vi "Query Channel Parameters.vi"(7 "Channel (1:Chan A)":i32(ring)=1 items=["Channel A"=1, "Channel B"=2, "Channel C"=3, "Channel D"=4, "Channel E"=5, "Channel F"=6, "Channel G"=7, "Channel H"=8], 8 "error in (no error)":errorcluster, 11 "VISA resource name":refnum<visa-resource-name>) -> (0 "error out":errorcluster, 2 "Chan Parameters":T1={"Channel"=1, "Chan State"=TRUE, "Chan Sync Source"=0, "Chan Gate Logic"=enum."Disabled", "Chan Mode"=enum."Normal", "Chan Wait #"=-1, "Chan Delay"=nan, "Chan Width"=nan, "Chan Burst #"=-1, "Chan DC On"=-1, "Chan DC Off"=-1, "Chan Polarity"=FALSE, "Chan MUX Value"=-1, "Chan Level Out"=enum."TTL", "Chan Lev Adjust"=0.0, "Chan Gate Mode"=enum."Disabled"} {"Chan Sync Source" items=["System (To)", "Channel A", "Channel B", "Channel C", "Channel D", "Channel E", "Channel F", "Channel G", "Channel H"]; "Chan Width" format="%.3p"; "Chan Delay" format="%.3p"; "Chan Lev Adjust" format="%.3p"; "Channel" items=["Channel A"=1, "Channel B"=2, "Channel C"=3, "Channel D"=4, "Channel E"=5, "Channel F"=6, "Channel G"=7, "Channel H"=8]}, 3 "VISA resource name out":refnum<visa-resource-name>)   [LabVIEW 2013]
doc: "This VI reads all channel parameters for the selected channel."
uses:
  Channel Parameters.ctl
  Berkeley Nucleonics 500 Series.lvlib
panel:
  # "Input"
  # "Normal\nSingle\nBurst"
  # "Burst"
  # "Duty Cycle"
  # "Output"
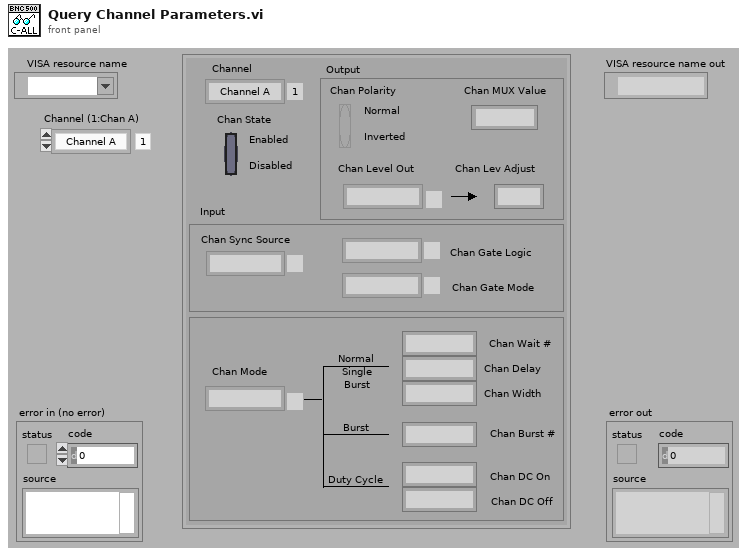
[diagram p1: front panel]
types:
  T1 = typedef "Channel Parameters.ctl" = cluster{"Channel":i32, "Chan State":bool, "Chan Sync Source":i32, "Chan Gate Logic":enum16{"Disabled", "Low", "High"}, "Chan Mode":enum16{"Normal", "Single", "Burst", "Duty Cycle"}, "Chan Wait #":i32, "Chan Delay":dbl, "Chan Width":dbl, "Chan Burst #":i32, "Chan DC On":i32, "Chan DC Off":i32, "Chan Polarity":bool, "Chan MUX Value":i32, "Chan Level Out":enum16{"TTL", "Adjustable", "35 Volt", "Optical"}, "Chan Lev Adjust":dbl, "Chan Gate Mode":enum16{"Disabled", "Pulse Inhibit", "Output Inhibit"}}
  T2 = cluster{"Gate Logic":enum16{"Disabled", "Low", "High"}, "Sync Source":i32, "Gate Mode":enum16{"Disabled", "Pulse Inhibit", "Output Inhibit"}}
  T3 = enum16{"Disabled", "Pulse Inhibit", "Output Inhibit"}
  T4 = cluster{"Mode":enum16{"Normal", "Single", "Burst", "Duty Cycle"}, "Burst #":i32, "DC Off":i32, "DC On":i32, "Delay":dbl, "Width":dbl, "Wait #":i32}
  T5 = enum16{"Normal", "Single", "Burst", "Duty Cycle"}
  T6 = cluster{"Polarity Out":bool, "Level Value":dbl, "Level Out":enum16{"TTL", "Adjustable", "35 Volt", "Optical"}, "MUX Value":i32}
  T7 = enum16{"TTL", "Adjustable", "35 Volt", "Optical"}
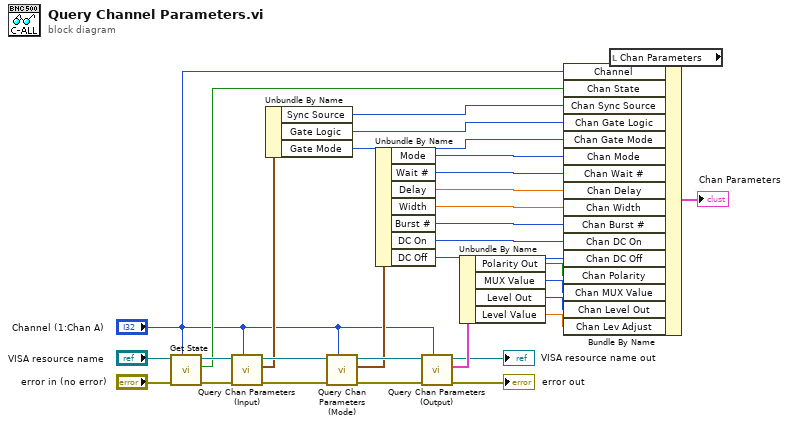
[diagram p0: block diagram]
diagram:
  n1 = call "Get State.vi"("Channel (1: Chan A)"="Channel (1:Chan A)", "error in (no error)"="error in (no error)", "VISA resource name"="VISA resource name") -> ("error out"=w26:errorcluster, "State"=w23:bool, "VISA resource name out"=w27:refnum<visa-resource-name>)  [unwired: 6 in]
  n2 = call "Query Chan Parameters (Input).vi"("Channel (1: Chan A)"="Channel (1:Chan A)", "error in (no error)"=w26, "VISA resource name"=w27) -> ("error out"=w30:errorcluster, "Input Parameters"=w22:T2, "VISA resource name out"=w31:refnum<visa-resource-name>)  [unwired: 6 in]
  n3 = Unbundle By Name(w22) -> ("Sync Source"=w21:i32, "Gate Logic"=w20:enum16{"Disabled", "Low", "High"}, "Gate Mode"=w2:T3)
  n4 = call "Query Chan Parameters (Mode).vi"("Channel (1: Chan A)"="Channel (1:Chan A)", "error in (no error)"=w30, "VISA resource name"=w31) -> ("error out"=w29:errorcluster, "Mode Parameters"=w19:T4, "VISA resource name out"=w28:refnum<visa-resource-name>)  [unwired: 6 in]
  n5 = Unbundle By Name(w19) -> ("Mode"=w18:T5, "Wait #"=w17:i32, "Delay"=w15:dbl, "Width"=w16:dbl, "Burst #"=w14:i32, "DC On"=w13:i32, "DC Off"=w12:i32)
  n6 = call "Query Chan Parameters (Output).vi"("Channel (1: Chan A)"="Channel (1:Chan A)", "error in (no error)"=w29, "VISA resource name"=w28) -> ("error out"=→"error out":errorcluster, "Output Parameters"=w11:T6, "VISA resource name out"=→"VISA resource name out":refnum<visa-resource-name>)  [unwired: 6 in]
  n7 = Unbundle By Name(w11) -> ("Polarity Out"=w10:bool, "MUX Value"=w9:i32, "Level Out"=w8:T7, "Level Value"=w7:dbl)
  n8 = local read "Chan Parameters"() -> (w3:T1)
  n9 = Bundle By Name(cluster=w3, "Channel"="Channel (1:Chan A)", "Chan State"=w23, "Chan Sync Source"=w21, "Chan Gate Logic"=w20, "Chan Gate Mode"=w2, "Chan Mode"=w18, "Chan Wait #"=w17, "Chan Delay"=w15, "Chan Width"=w16, "Chan Burst #"=w14, "Chan DC On"=w13, "Chan DC Off"=w12, "Chan Polarity"=w10, "Chan MUX Value"=w9, "Chan Level Out"=w8, "Chan Lev Adjust"=w7) -> (→"Chan Parameters":T1)
